vi "Chamber controller March 30 2017.vi"() -> ()   [LabVIEW 2014]
uses:
  <vilib>/Instr/_visa.llb/VISA Configure Serial Port (Instr).vi
  Environmental Chamber LabVIEW and Instruments/Drivers and Software/Keithley 2100 Series/Public/Configure/Configure 2 Wire Resistance.vi
  <vilib>/Utility/file.llb/Write To Spreadsheet File (string).vi
  <vilib>/Utility/file.llb/Read From Spreadsheet File (string).vi
  Environmental Chamber LabVIEW and Instruments/Drivers and Software/keithley_6430/Keithley 6430/Public/Data/Read (Single Point).vi
  Environmental Chamber LabVIEW and Instruments/Drivers and Software/LabVIEW 8.2 Drivers/keithley_24xx/Keithley 24XX/Public/Data/Read (Single Point).vi
  Environmental Chamber LabVIEW and Instruments/Drivers and Software/keithley_24xx/Keithley 24XX/Keithley 24XX.lvlib
  Environmental Chamber LabVIEW and Instruments/Drivers and Software/keithley_6430/Keithley 6430/Keithley 6430.lvlib
  Environmental Chamber LabVIEW and Instruments/Drivers and Software/Keithley 2100 Series/Keithley 2100 Series.lvlib
panel:
  in  "points":i32=10
  in  "average points?":bool
  in  "Pressure parameters cluster":T1={"valve % open"=0.0, "Desired pressure"=0.0, "Vapor sccm"=0.0, "Gas sccm"=0.0, "Valve mode"=enum."% Open", "Pressure Mode"=enum."Abs. pressure", "analyte partial pressure"=23.8, "Turbo pump\nauto on"=TRUE, "Valve position (%)"=0.0, "read pressure"=0.0, "read vapor flow"=0.0, "read gas flow"=0.0} caption="Pressure settings" {"read gas flow" format="%#_3g"; "read vapor flow" format="%#_3g"; "read pressure" format="%#_7f"; "Valve position (%)" format="%#_3g"; "analyte partial pressure" min=0.0 max=100.0 step=5.0; "Gas sccm" min=0 max=200 step=5; "Vapor sccm" min=0 max=200 step=5; "Desired pressure" min=0.0 max=760.0 step=5.0; "valve % open" min=0.0 max=100.0 step=5.0 format="%#_2f"}
  out "pressure chart":cluster{"pressure":dbl}(graph)
  out "arduino qcm stack plot":T2(graph)
  in  "K-2420 tab control":enum32{"K-2420 Measure", "K-2420 Apply bias"}(tab)
  out "K-2420 2":cluster{"Resistance":sgl}(graph)
  in  "Bias (V)":dbl min=-5.0 max=5.0 step=5e-06
  out "K-2420 4":cluster{"Applied Voltage (V)":dbl}(graph)
  out "saving data?":bool
  in  "Data logging settings":T3={"Save during sequence only"=TRUE, "Save now"=FALSE, "sec between points"=0.0, "Current data file path"=path "", "Save sample/gas names"={"QCM1"="", "QCM2"="", "QCM3"="", "QCM4"="", "QCM5"="NOT WORKING", "QCM6"="", "SRS"="bareAu", "K-2420"="", "K-6430"="", "K-2100"="", "Gas"="NOT WORKING", "Vapor"="CO2"}, "add notes to file"=FALSE} {"sec between points" min=0.0 max=30.0 format="%#_13g"}
  in  "Sequence cluster":T4={"Save sequence"=FALSE, "Clear sequence"=FALSE, "Import sequence file"=FALSE, "Run Sequence"=FALSE, "Stop program when sequence ends"=TRUE, "User-defined\nsequence"=[], "Sequence end time"="", "Sequence\npreview"=[], "Current\nstep"=0, "Display"=0, "Sequence length (hrs)"=0.0} caption="Pressure settings" {"Display" items=["pressure", "gas flow", "vapor flow", "bias"]}
  out "J-KEM temp chart":dbl(graph)
  out "State date/time":string caption="Start time"
  out "K-2100 (Ohm)":cluster{"Measurement":dbl}(graph) caption="K-2100"
  out "K-6430":cluster{"Measurement":dbl}(graph)
  in  "Gate time (s)":enum16{"0.1", "1.0 ", "10"}(ring)=enum."1.0 "
  out "Hz":dbl format="%#.7f"
  out "QCM plot":T5(graph)
  in  "Stop":bool
  in  "Clear all charts":bool
  out "O2 sensor output":dbl[](array[numeric]) caption="atm\nTorr"
  in  "rapidox O2 Sensor":bool
  in  "setnag O2 Pump":bool
  in  "Baud Rate 2":i32(ring)=2 items=["2400", "4800", "9600", "19200", "38400", "57600", "115200"]
  in  "Com Port":i32(ring) items=["Com 1", "Com 2", "Com 3", "Com 4", "Com 5", "Com 6", "COM 7", "COM 8", "COM 9", "COM 10", "COM 11", "COM 12", "com 13", "COM 14"]
  in  "Com Port 2":i32(ring) items=["Com 1", "Com 2", "Com 3", "Com 4", "Com 5", "Com 6", "COM 7", "COM 8", "COM 9", "COM 10", "COM 11", "COM 12", "com 13", "COM 14"]
  out "Waveform Chart":cluster{dbl}(graph)
  out "O2 Concentration (PPM)":dbl
  out "Waveform Chart 6":cluster{dbl}(graph)
  # "SRS"
  # "Currently Unused"
  # "100%"
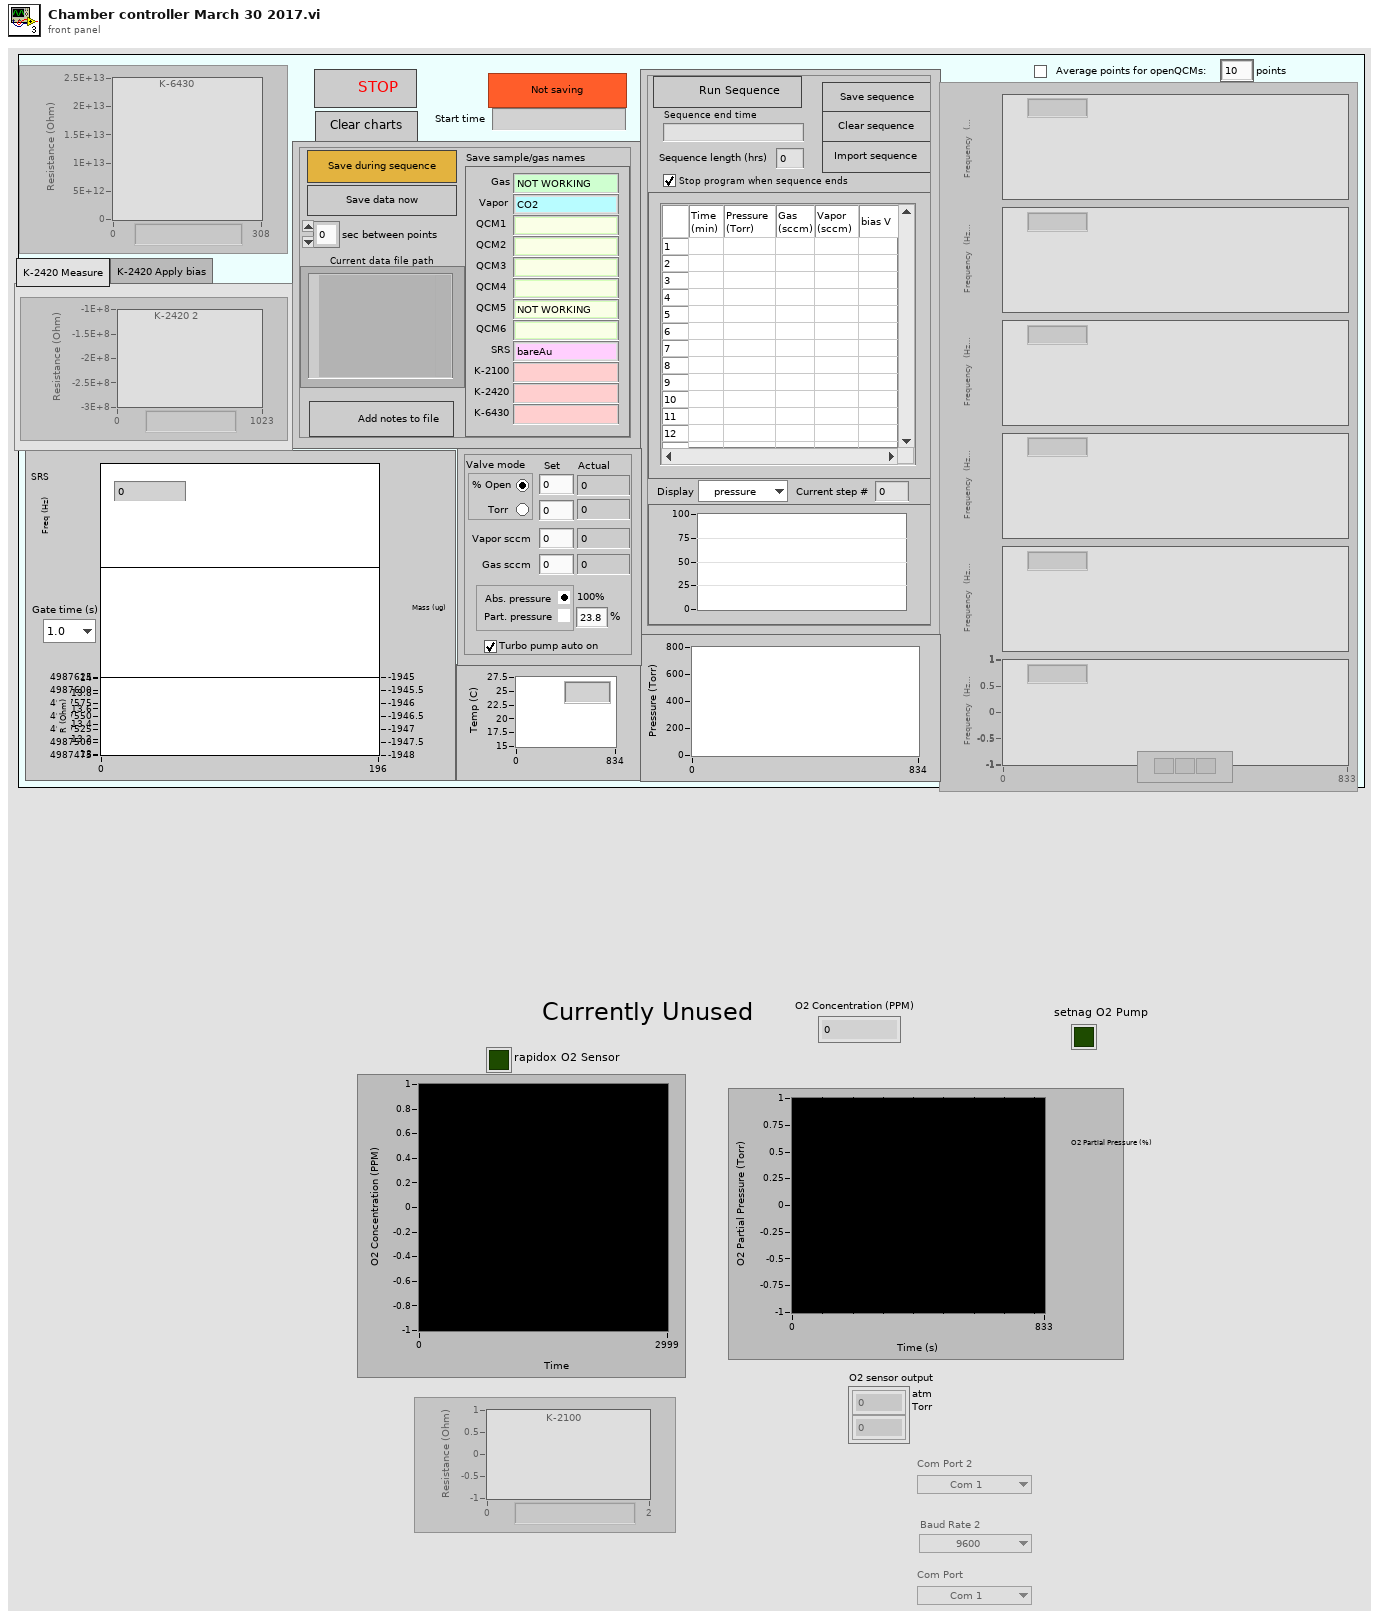
[diagram p1: front panel]
types:
  T1 = cluster{"valve % open":dbl, "Desired pressure":dbl, "Vapor sccm":sgl, "Gas sccm":sgl, "Valve mode":enum32{"% Open", "Torr "}, "Pressure Mode":enum32{"Abs. pressure", " Part. pressure"}, "analyte partial pressure":dbl, "Turbo pump\nauto on":bool, "Valve position (%)":dbl, "read pressure":dbl, "read vapor flow":dbl, "read gas flow":dbl}
  T2 = cluster{"mean":dbl, "mean":dbl, "mean":dbl, "mean":dbl, "mean":dbl, "mean":dbl}
  T3 = cluster{"Save during sequence only":bool, "Save now":bool, "sec between points":dbl, "Current data file path":path, "Save sample/gas names":cluster{"QCM1":string, "QCM2":string, "QCM3":string, "QCM4":string, "QCM5":string, "QCM6":string, "SRS":string, "K-2420":string, "K-6430":string, "K-2100":string, "Gas":string, "Vapor":string}, "add notes to file":bool}
  T4 = cluster{"Save sequence":bool, "Clear sequence":bool, "Import sequence file":bool, "Run Sequence":bool, "Stop program when sequence ends":bool, "User-defined\nsequence":string[][], "Sequence end time":string, "Sequence\npreview":cluster{dbl[], dbl[]}[], "Current\nstep":i32, "Display":u16, "Sequence length (hrs)":dbl}
  T5 = cluster{"Frequency out":dbl, "Numeric Control":dbl, "Resistance out":dbl}
  T6 = cluster{"Keithley 6430":bool, "J-KEM":bool, "Keithley 2420":bool, "Keithley 2100":bool, "SRS QCM":bool, "Pressure control":bool, "Arduino":bool}
  T7 = cluster{"Arduino 1":refnum<visa-resource-name>, "Arduino 2":refnum<visa-resource-name>, "Arduino 3":refnum<visa-resource-name>, "Arduino 4":refnum<visa-resource-name>, "Arduino 5":refnum<visa-resource-name>, "Arduino 6":refnum<visa-resource-name>}
  T8 = enum8{"Enabled", "Disabled", "Disabled and Grayed Out"}
  T9 = enum16{"open", "open or create", "create or replace", "create", "open (read only)"}
  T10 = enum16{"no parity", "odd parity", "even parity", "mark parity", "space parity"}
  T11 = cluster{"mean":dbl, "mean":dbl, "mean":dbl, "mean":dbl, "mean":dbl, "mean":dbl}[]
  T12 = cluster{"Frequency out":dbl, "Numeric Control":dbl, "Resistance out":dbl}[]
  T13 = cluster{"String":string, "String":string, "String":string}
  T14 = cluster{bool, "task out":refnum<k21>, "error out":errorcluster, "task out":refnum<k21>, "error out":errorcluster, "turbo pump":refnum<visa-resource-name>, "error out":errorcluster}
  T15 = cluster{bool, "task out":refnum<k21>, "error out":errorcluster, "task out":refnum<k21>, "error out":errorcluster, "VISA resource name out":refnum<visa-resource-name>, "error out":errorcluster}
  T16 = cluster{bool, "VISA resource name":refnum<visa-resource-name>, "error out":errorcluster}
  T17 = cluster{bool, "VISA resource name out":refnum<visa-resource-name>, "error out":errorcluster}
  T18 = cluster{"VISA resource name out":refnum<visa-resource-name>, "error out":errorcluster, "VISA resource name out":refnum<visa-resource-name>, "error out":errorcluster, "VISA resource name out":refnum<visa-resource-name>, "error out":errorcluster, "VISA resource name out":refnum<visa-resource-name>, "error out":errorcluster, "VISA resource name out":refnum<visa-resource-name>, "error out":errorcluster, "VISA resource name out 2":refnum<visa-resource-name>, "error out 2":errorcluster}
  T19 = cluster{"Boolean":bool, "VISA resource name out":refnum<visa-resource-name>, "error out":errorcluster}
  T20 = cluster{bool, "VISA out":refnum<visa-resource-name>, "error out":errorcluster}
  T21 = cluster{"Boolean":bool, "VISA out":refnum<visa-resource-name>, "error out":errorcluster}
  T22 = cluster{"Numeric Control":dbl, "Cluster":cluster{"Numeric Control":dbl}, "String":string, "error out":errorcluster}
  T23 = cluster{bool, "Com Port":i32, "Numeric Control out":dbl}
  T24 = cluster{"Arduino address":refnum<visa-resource-name>, "error in (no error)":errorcluster, "Arduino address 2":refnum<visa-resource-name>, "error in (no error) 2":errorcluster, "Arduino address 3":refnum<visa-resource-name>, "error in (no error) 3":errorcluster, "Arduino address 4":refnum<visa-resource-name>, "error in (no error) 4":errorcluster, "Arduino address 5":refnum<visa-resource-name>, "error in (no error) 5":errorcluster, "Arduino address 6":refnum<visa-resource-name>, "error in (no error) 6":errorcluster}
  T25 = cluster{"String":string, "String":string, "String":string, "String":string, "String":string, "String":string}
  T26 = cluster{"valve % open":dbl, "Desired pressure":dbl, "Vapor sccm":sgl, "Gas sccm":sgl, "Valve mode":enum32{"% Open", "Torr "}, "Pressure Mode":enum32{"Abs. pressure", " Part. pressure"}, "analyte partial pressure":dbl}
  T27 = cluster{"User-defined\nsequence":string[][], "Present (s)":dbl, "current  step # in":i32, "sequence end time in":timestamp}
  T28 = cluster{"current  step # in":i32, "sequence end time in":timestamp, "Boolean":bool}
  T29 = cluster{"press/RH/gas/vapor":cluster{"pressure":string, "RH":string, "gas flow":string, "vapor flow":string}, "Cluster":cluster{"Valve position (%)":dbl, "read pressure":dbl, "read vapor flow":dbl, "read gas flow":dbl}}
  T30 = cluster{"Boolean":bool, "task out":refnum<k21>, "error out":errorcluster, "task out":refnum<k21>, "error out":errorcluster, "VISA resource name out":refnum<visa-resource-name>, "error out":errorcluster}
  T31 = cluster{"String":dbl, "String":dbl, "String":dbl, "String":dbl, "String":dbl, "String":dbl}
  T32 = cluster{"pressure":string, "RH":string, "gas flow":string, "vapor flow":string}
  T33 = cluster{"Valve position (%)":dbl, "read pressure":dbl, "read vapor flow":dbl, "read gas flow":dbl}
  T34 = cluster{"f":dbl, "f":dbl, "f":dbl, "f":dbl, "f":dbl}[]
  T35 = cluster{"QCM1":string, "QCM2":string, "QCM3":string, "QCM4":string, "QCM5":string, "QCM6":string, "SRS":string, "K-2420":string, "K-6430":string, "K-2100":string, "Gas":string, "Vapor":string}
  T36 = cluster{"String data out":string, string, string, string}
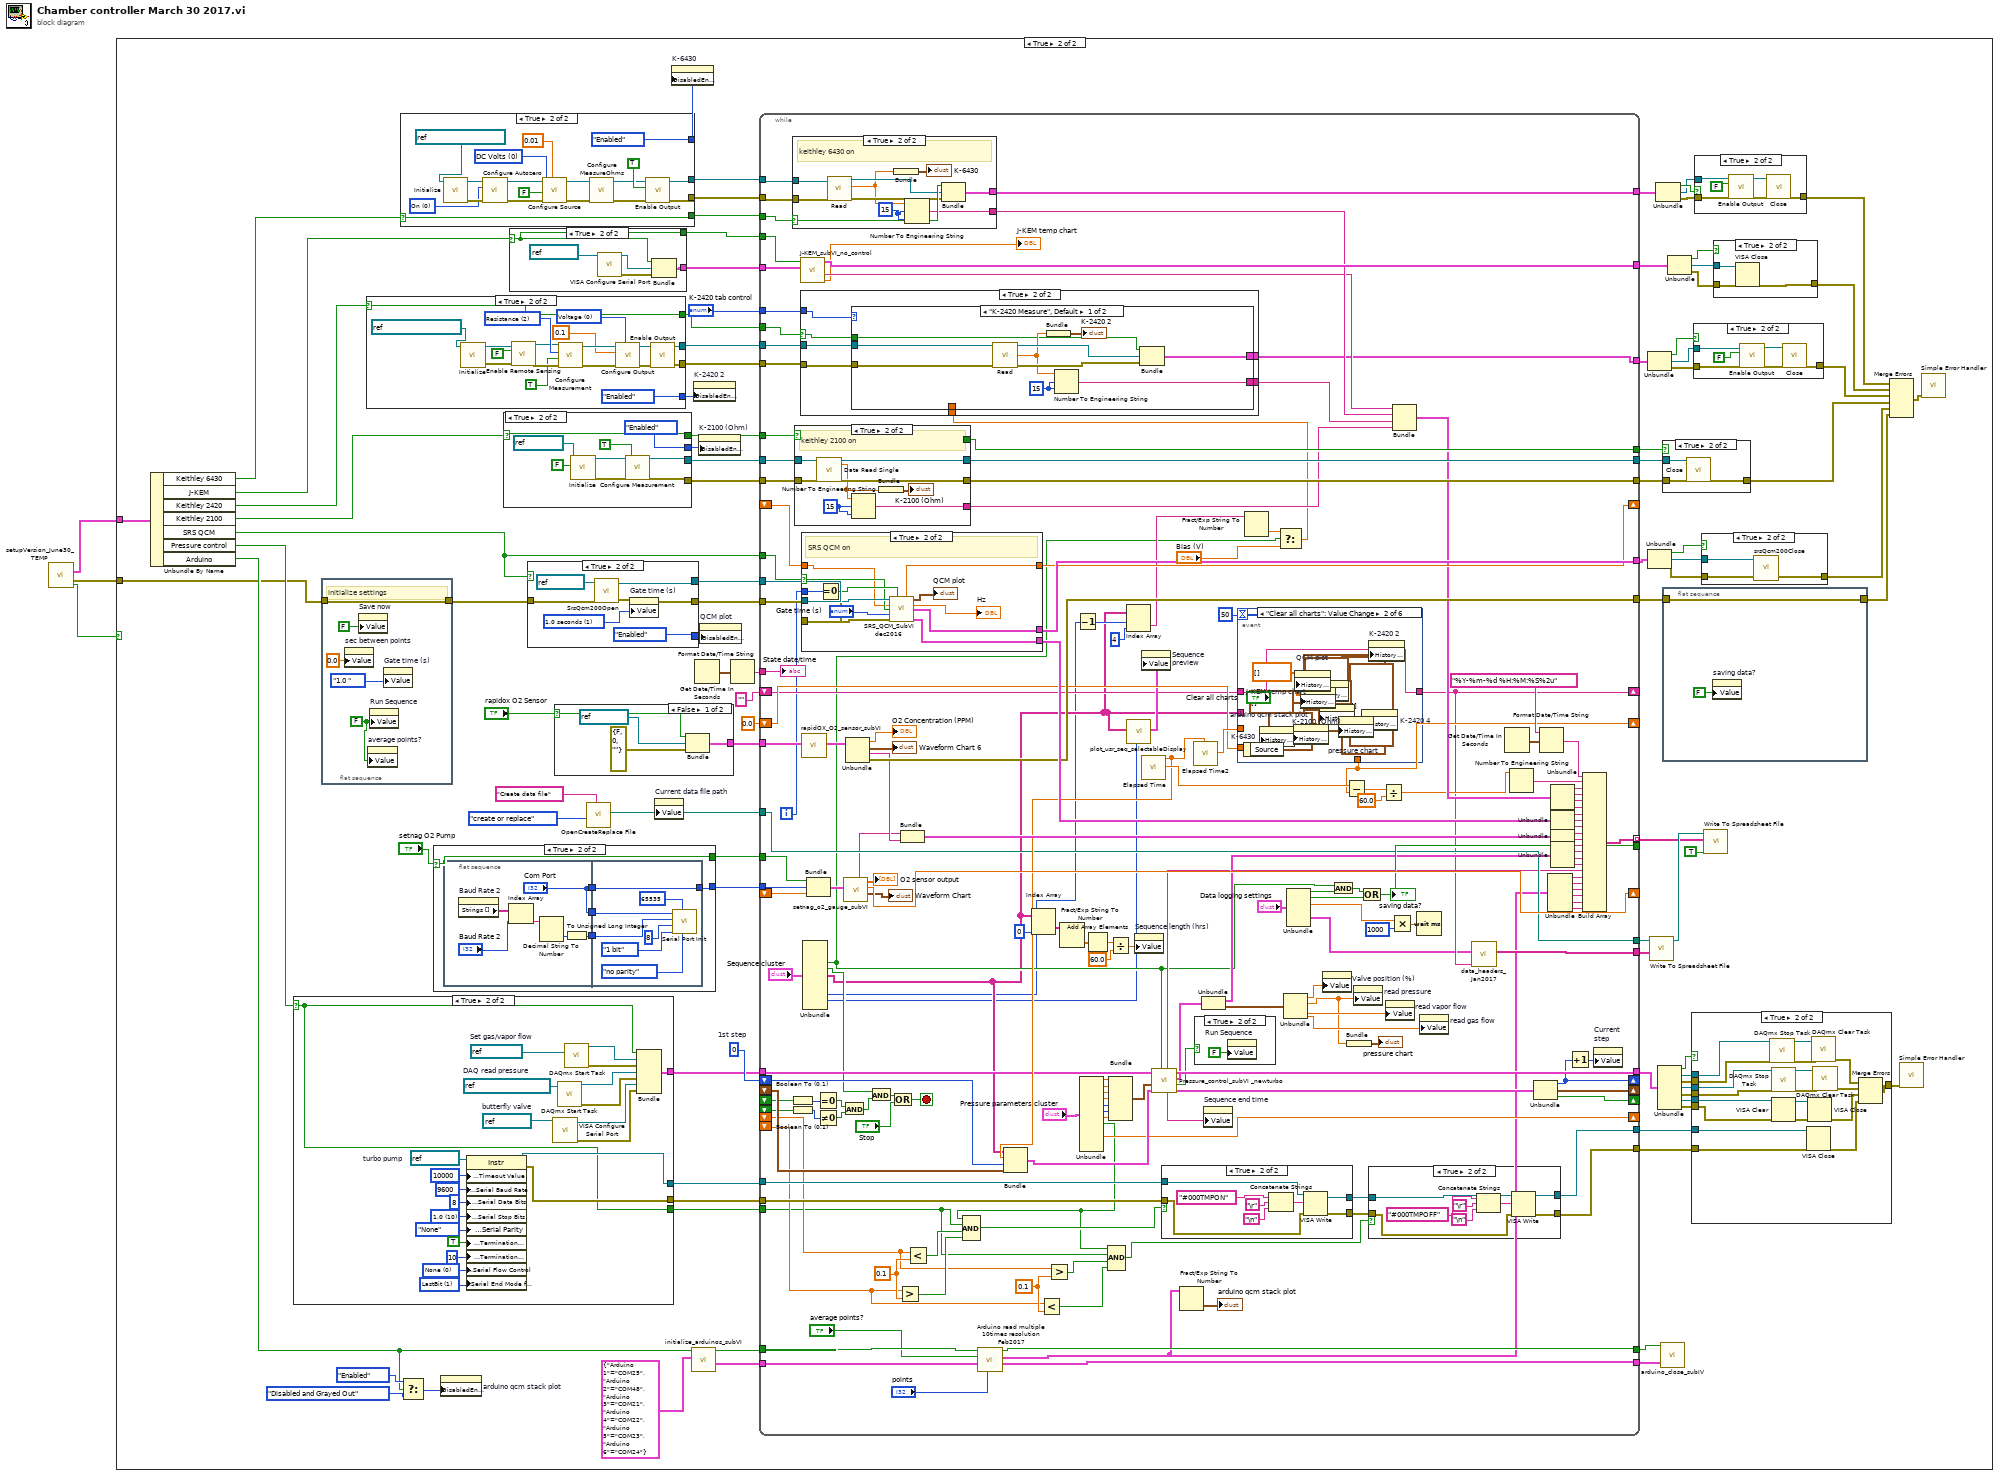
[diagram p0: block diagram]
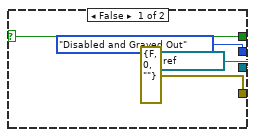
[diagram p4: hidden frame]
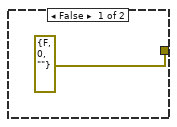
[diagram p5: hidden frame]
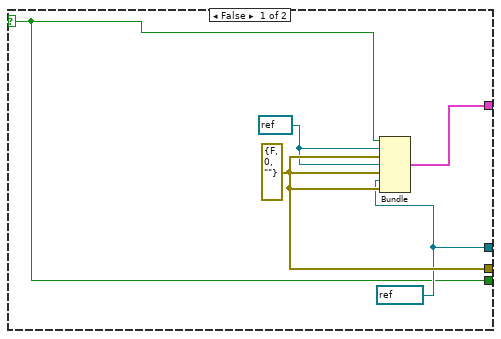
[diagram p6: hidden frame]
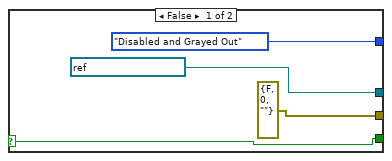
[diagram p8: hidden frame]
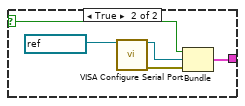
[diagram p9: hidden frame]
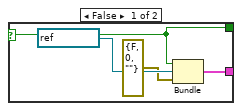
[diagram p11: hidden frame]
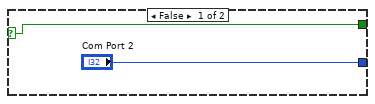
[diagram p12: hidden frame]
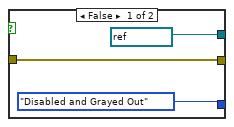
[diagram p14: hidden frame]
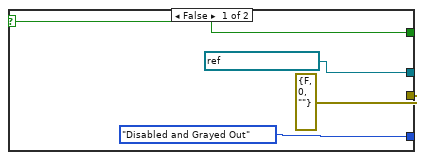
[diagram p16: hidden frame]
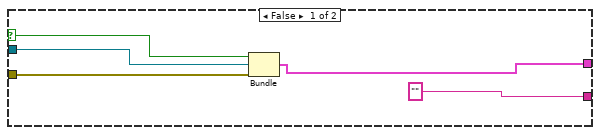
[diagram p17: hidden frame]
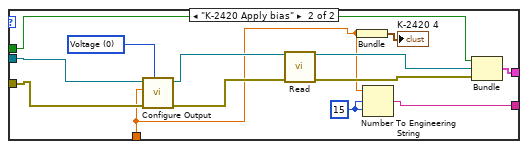
[diagram p18: hidden frame]
diagram:
  n1 = call "setupVersion_June30_TEMP.vi"() -> ("Instruments on/off"=w1:T6, "error IO"=w2:errorcluster, "OK"=w3:bool)  [unwired: 13 in]
  n2 = case shown="True" w3 {
    tunnel: w2 -> [_ w22]
    tunnel: w1 -> [_ w32]
    frame False {
    }
    frame True {
      w38 = 0  # 1st step
      n3 = Unbundle By Name(w32) -> ("Keithley 6430"=w31:bool, "J-KEM"=w30:bool, "Keithley 2420"=w29:bool, "Keithley 2100"=w28:bool, "SRS QCM"=w27:bool, "Pressure control"=w26:bool, "Arduino"=w25:bool)
      n4 = case shown="True" w26 {
        selector: w26 -> [w144 w149]
        tunnel: [w148 w150] -> w20
        tunnel: [w147 w152] -> w12
        tunnel: [w145 w151] -> w13
        tunnel: [w144 w149] -> w11
        frame False {
          w145 = refnum<visa-resource-name> refnum ("turbo pump")
          w146 = refnum<k21> refnum ("task out")
          w147 = errorcluster {"status"=FALSE, "code"=0, "source"=""} ("error out")
          n5 = Bundle(w144, "task out"=w146, "error out"=w147, "task out"=w146, "error out"=w147, "turbo pump"=w145, "error out"=w147) -> (w148:T14)  [unwired: 1 in]
        }
        frame True {
          w156 = u16 1 items=["None", "LastBit", "TermChar"] ("Serial Settings:Serial End Mode for Reads")
          w154 = u16 0 items=["None", "XON/XOFF", "RTS/CTS", "XON/XOFF & RTS/CTS", "DTR/DSR", "XON/XOFF & DTR/DSR"] ("flow control (0:none)")
          w157 = u16 10 items=["1.0"=10, "1.5"=15, "2.0"=20] ("stop bits (10: 1 bit)")
          w153 = refnum<visa-resource-name> "COM7"  # turbo pump
          w169 = refnum<visa-resource-name> "COM5"  # butterfly valve
          w170 = refnum<k21> "Setflow"  # Set gas/vapor flow
          w171 = refnum<k21> "AllDaqReadings"  # DAQ read pressure
          n6 = property class="Instr"(reference=w153, "General Settings:Timeout Value"=u32 10000 ("timeout (10sec)"), "Serial Settings:Serial Baud Rate"=u32 9600 ("baud rate (9600)"), "Serial Settings:Serial Data Bits"=u16 8 ("data bits (8)"), "Serial Settings:Serial Stop Bits"=w157, "Serial Settings:Serial Parity"=enum16{"None", "Odd", "Even", "Mark", "Space"}."None" ("parity (0:none)"), "Message Based Settings:Termination Character Enable"=TRUE ("Enable Termination\nChar (T)"), "Message Based Settings:Termination Character"=u8 10 ("termination char\n(0xA = '\\n' = LF)"), "Serial Settings:Serial Flow Control"=w154, "Serial Settings:Serial End Mode for Reads"=w156) -> (reference out=w151:refnum<visa-resource-name>, error out=w152:errorcluster)  [unwired: 1 in]
          n7 = call-poly "VISA Configure Serial Port"("VISA resource name"=w169) -> ("VISA resource name out"=w164:refnum<visa-resource-name>, "error out"=w163:errorcluster)  [unwired: 13 in]
          n8 = call <vilib>:"DAQmx Start Task.vi"("task/channels in"=w171) -> ("task out"=w166:refnum<k21>, "error out"=w165:errorcluster)  [unwired: 13 in]
          n9 = call <vilib>:"DAQmx Start Task.vi"("task/channels in"=w170) -> ("task out"=w168:refnum<k21>, "error out"=w167:errorcluster)  [unwired: 13 in]
          n10 = Bundle(w149, "task out"=w168, "error out"=w167, "task out"=w166, "error out"=w165, "VISA resource name out"=w164, "error out"=w163) -> (w150:T15)  [unwired: 1 in]
        }
      }
      n11 = flat-sequence {
        tunnel: [w101] -> w21
        tunnel: w22 -> [w101]
        frame #0 {
          w100 = FALSE ("Value")
          # "initialize settings"
          n12 = property on="sec between points" class="DigNum (strict)"("Value"=0.0) -> ()  [unwired: 2 in, 2 out]
          n13 = property on="Save now" class="Bool (strict)"("Value"=FALSE) -> ()  [unwired: 2 in, 2 out]
          n14 = property on="average points?" class="Bool (strict)"("Value"=w100) -> ()  [unwired: 2 in, 2 out]
          n15 = property on="Run Sequence" class="Bool (strict)"("Value"=w100) -> ()  [unwired: 2 in, 2 out]
          n16 = property on="Gate time (s)" class="Enum (strict)"("Value"=enum16{"0.1", "1.0 ", "10"}."1.0 " ("Gate time (sec)")) -> ()  [unwired: 2 in, 2 out]
        }
      }
      n17 = case shown="True" w29 {
        selector: w29 -> [w264 w268]
        tunnel: [refnum<visa-resource-name> "GPIB1::24::INSTR" ("VISA resource name") w277] -> w97
        tunnel: [errorcluster {"status"=FALSE, "code"=0, "source"=""} ("error out") w272] -> w96
        tunnel: [T8."Disabled and Grayed Out" ("Disabled") T8."Enabled" ("Disabled")] -> w4
        tunnel: [w264 w268] -> w54
        frame False {
        }
        frame True {
          w279 = u16 0 items=["Voltage", "Current"] ("Source Mode  (0: Voltage)")
          w284 = u16 2 items=["Volts", "Current", "Resistance"] ("Function (0: Volts)")
          n18 = call "Initialize.vi"("VISA resource name"=refnum<visa-resource-name> "GPIB1::24::INSTR") -> ("error out"=w273:errorcluster, "VISA resource name out"=w276:refnum<visa-resource-name>)  [unwired: 9 in]
          n19 = call "Enable Remote Sensing.vi"("error in (no error)"=w273, "Enable Remote Sensing (T: Enable)"=FALSE ("4-wire?"), "VISA resource name"=w276) -> ("error out"=w274:errorcluster, "VISA resource name out"=w275:refnum<visa-resource-name>)  [unwired: 7 in]
          n20 = call "Configure Measurement.vi"("error in (no error)"=w274, "Enable Auto Range (T:Enable)"=TRUE, "Function (0: Volts)"=w284, "VISA resource name"=w275) -> ("error out"=w283:errorcluster, "VISA resource name out"=w282:refnum<visa-resource-name>)  [unwired: 6 in]
          n21 = call "Configure Output.vi"("Source Mode  (0: Voltage)"=w279, "error in (no error)"=w283, "Output Level (0)"=0.1 ("Applied Voltage (V)"), "VISA resource name"=w282) -> ("error out"=w281:errorcluster, "VISA resource name out"=w280:refnum<visa-resource-name>)  [unwired: 6 in]
          n22 = call "Enable Output.vi"("error in (no error)"=w281, "VISA resource name"=w280) -> ("error out"=w272:errorcluster, "VISA resource name out"=w277:refnum<visa-resource-name>)  [unwired: 8 in]
        }
      }
      n23 = case shown="True" w31 {
        selector: w31 -> [w179 w184]
        tunnel: [refnum<visa-resource-name> "GPIB0::29::INSTR" ("VISA resource name") w195] -> w66
        tunnel: [errorcluster {"status"=FALSE, "code"=0, "source"=""} ("error out") w196] -> w65
        tunnel: [T8."Disabled and Grayed Out" ("Disabled") T8."Enabled" ("Disabled")] -> w60
        tunnel: [w179 w184] -> w53
        frame False {
        }
        frame True {
          w185 = u16 0 items=["DC Volts", "DC Current"] ("Source Function (0: DC Volts)")
          w192 = u16 0 items=["On", "Off", "Once"] ("Autozero  (0: On)")
          n24 = call "Initialize.vi"("VISA resource name"=refnum<visa-resource-name> "GPIB2::19::INSTR") -> ("error out"=w193:errorcluster, "VISA resource name out"=w194:refnum<visa-resource-name>)  [unwired: 4 in, 5 out]
          n25 = call "Configure Autozero.vi"("error in (no error)"=w193, "Autozero  (0: On)"=w192, "VISA resource name"=w194) -> ("error out"=w188:errorcluster, "VISA resource name out"=w190:refnum<visa-resource-name>)  [unwired: 7 in]
          n26 = call "Configure Source.vi"("V-Source Level [V]"=0.01, "error in (no error)"=w188, "Auto Range (T:Enable)"=FALSE, "Source Function (0: DC Volts)"=w185, "VISA resource name"=w190) -> ("error out"=w187:errorcluster, "VISA resource name out"=w189:refnum<visa-resource-name>)  [unwired: 5 in]
          n27 = call "Configure MeasureOhms.vi"("error in (no error)"=w187, "VISA resource name"=w189) -> ("error out"=w200:errorcluster, "VISA resource name out"=w198:refnum<visa-resource-name>)  [unwired: 4 in, 4 out]
          n28 = call "Enable Output.vi"("error in (no error)"=w200, "Enable Output (F:Off)"=TRUE ("Output (F:Off)"), "VISA resource name"=w198) -> ("error out"=w196:errorcluster, "VISA resource name out"=w195:refnum<visa-resource-name>)  [unwired: 7 out]
        }
      }
      n29 = Select(t=T8."Enabled" ("Disabled"), s=w25, f=T8."Disabled and Grayed Out" ("Disabled")) -> (s? t:f=w6:T8)
      n30 = case shown="True" "setnag O2 Pump" {
        selector: "setnag O2 Pump" -> [w223 w225]
        tunnel: ["Com Port 2" w226] -> w93
        tunnel: [w223 w225] -> w43
        frame False {
        }
        frame True {
          n31 = flat-sequence {
            tunnel: ["Com Port"] -> w229
            tunnel: [w231] -> w228
            tunnel: ["Com Port"] -> w227
            tunnel: w229 -> [w237]
            tunnel: w228 -> [w236]
            tunnel: w227 -> [w238]
            tunnel: [w238] -> w226
            frame #0 {
              n32 = property on="Baud Rate 2" class="Ring (strict)"() -> ("Strings []"=w233:string[])  [unwired: 2 in, 2 out]
              n33 = Index Array(array=w233, index="Baud Rate 2") -> (element=w234:string)
              n34 = Decimal String To Number(string=w234) -> (number=w232:i32)  [unwired: 2 in, 1 out]
              n35 = To Unsigned Long Integer(number=w232) -> (unsigned 32bit integer=w231:u32)
            }
            frame #1 {
              n36 = call <vilib>:"Serial Port Init.vi"("parity"=T10."no parity", "buffer size"=u16 65535, "stop bits"=enum16{"1 bit", "1.5 bits", "2 bits"}."1 bit", "data bits"=u16 8, "baud rate"=w236, "port number"=w237) -> ()  [unwired: 1 in, 1 out]
            }
          }
        }
      }
      n37 = property on="arduino qcm stack plot" class="WFChart (strict)"("DisabledEnum"=w6) -> ()  [unwired: 2 in, 2 out]
      n38 = case shown="True" w28 {
        selector: w28 -> [w112 w117]
        tunnel: [refnum<visa-resource-name> "K-2100" ("VISA resource name out") w120] -> w52
        tunnel: [errorcluster {"status"=FALSE, "code"=0, "source"=""} ("error out") w119] -> w51
        tunnel: [w112 w117] -> w50
        tunnel: [T8."Disabled and Grayed Out" ("Disabled") T8."Enabled" ("Disabled")] -> w45
        frame False {
        }
        frame True {
          n39 = call "Initialize.vi"("VISA resource name"=refnum<visa-resource-name> "K-2100", "Reset? (T: Reset)"=FALSE) -> ("VISA resource name out"=w121:refnum<visa-resource-name>, "error out"=w118:errorcluster)  [unwired: 16 in]
          n40 = call-poly "Configure Measurement.vi"("VISA resource name"=w121, "error in (no error)"=w118, "Auto Range? (T: Auto)"=TRUE) -> ("VISA resource name out"=w120:refnum<visa-resource-name>, "error out"=w119:errorcluster)  [unwired: 15 in]
        }
      }
      n41 = case shown="True" w30 {
        selector: w30 -> [w214 w219]
        tunnel: [w215 w220] -> w82
        tunnel: [w214 w219] -> w76
        frame False {
          n42 = Bundle(w214, "VISA resource name"=refnum<visa-resource-name> "COM3", "error out"=errorcluster {"status"=FALSE, "code"=0, "source"=""}) -> (w215:T16)  [unwired: 1 in]
        }
        frame True {
          n43 = call-poly "VISA Configure Serial Port"("VISA resource name"=refnum<visa-resource-name> "COM3") -> ("VISA resource name out"=w221:refnum<visa-resource-name>, "error out"=w218:errorcluster)  [unwired: 13 in]
          n44 = Bundle(w219, "VISA resource name out"=w221, "error out"=w218) -> (w220:T17)  [unwired: 1 in]
        }
      }
      n45 = case shown="True" w27 {
        tunnel: [refnum<visa-resource-name> "COM6" ("VISA in") w253] -> w95
        tunnel: [w248 w250] -> w94
        tunnel: w21 -> [w248 w255]
        tunnel: [T8."Disabled and Grayed Out" ("Disabled") T8."Enabled" ("Disabled")] -> w61
        frame False {
        }
        frame True {
          w252 = u16 1 items=["0.1 seconds", "1.0 seconds", "10.0 seconds"] ("Gate time")
          n46 = call "SrsQcm200Open.vi"("error in"=w255, "VISA in"=refnum<visa-resource-name> "COM6") -> ("error out"=w251:errorcluster, "VISA out"=w253:refnum<visa-resource-name>)  [unwired: 3 in]
          n47 = property on="Gate time (s)" class="Enum (strict)"(error in=w251, "Value"=w252) -> (error out=w250:errorcluster)  [unwired: 1 in, 1 out]
        }
      }
      n48 = case shown="False" "rapidox O2 Sensor" {
        selector: "rapidox O2 Sensor" -> [w201 w206]
        tunnel: [w202 w207] -> w72
        frame False {
          n49 = Bundle(w201, "VISA resource name"=refnum<visa-resource-name> "COM7", "error out"=errorcluster {"status"=FALSE, "code"=0, "source"=""}) -> (w202:T16)  [unwired: 1 in]
        }
        frame True {
          n50 = call-poly "VISA Configure Serial Port"("VISA resource name"=refnum<visa-resource-name> "COM7") -> ("VISA resource name out"=w208:refnum<visa-resource-name>, "error out"=w205:errorcluster)  [unwired: 13 in]
          n51 = Bundle(w206, "VISA resource name out"=w208, "error out"=w205) -> (w207:T17)  [unwired: 1 in]
        }
      }
      n52 = call "OpenCreateReplace File.vi"("prompt"="Create data file", "function (open:0)"=T9."create or replace") -> ("new file path"=w8:path)  [unwired: 6 in, 3 out]
      n53 = property on="Current data file path" class="Path"("Value"=w8) -> ()  [unwired: 2 in, 2 out]
      n54 = property on="K-6430" class="WFChart (strict)"("DisabledEnum"=w60) -> ()  [unwired: 2 in, 2 out]
      n55 = call "initialize_arduinos_subVI.vi"("arduino 1-6 addresses"=T7 {"Arduino 1"="COM25", "Arduino 2"="COM48", "Arduino 3"="COM21", "Arduino 4"="COM22", "Arduino 5"="COM23", "Arduino 6"="COM24"} ("Arduino COMs"), "arduinos on?"=w25) -> ("arduino addresses/errors"=w39:T18, "arduinos on/off"=w58:bool)  [unwired: 8 in]
      n56 = property on="K-2420 2" class="WFChart (strict)"("DisabledEnum"=w4) -> ()  [unwired: 2 in, 2 out]
      n57 = Get Date/Time In Seconds() -> (seconds since 1Jan1904=w99:timestamp)
      n58 = property on="K-2100 (Ohm)" class="WFChart (strict)"("DisabledEnum"=w45) -> ()  [unwired: 2 in, 2 out]
      n59 = property on="QCM plot" class="WFChart (strict)"("DisabledEnum"=w61) -> ()  [unwired: 2 in, 2 out]
      n60 = Format Date/Time String(seconds (now)=w99) -> (date/time string=w42:string)  [unwired: 2 in]
      n61 = while {
        shift-right: [w464] -> _
        shift-left: _ -> [w405]
        tunnel: [w452] -> w59 mode=indexing if=w426
        tunnel: w54 -> [w325]
        tunnel: w97 -> [w327]
        tunnel: w96 -> [w326]
        tunnel: w95 -> [w463]
        tunnel: w94 -> [w462]
        tunnel: w27 -> [w461]
        tunnel: w43 -> [w407]
        tunnel: w93 -> [w408]
        tunnel: [w320] -> w90
        tunnel: [w460] -> w86
        tunnel: w82 -> [w459]
        tunnel: [w458] -> w81
        tunnel: w76 -> [w457]
        tunnel: w72 -> [w415]
        tunnel: [w411] -> w24
        tunnel: [w356] -> w71
        tunnel: w8 -> [w356]
        shift-right: [w450] -> _
        shift-left: _ -> [w451]
        tunnel: w66 -> [w456]
        tunnel: w65 -> [w455]
        tunnel: [w454] -> w64
        tunnel: [w426] -> _
        tunnel: w58 -> [w298]
        tunnel: w39 -> [w299]
        tunnel: [w296] -> w56
        tunnel: [w295] -> w57
        tunnel: [w300] -> w55
        tunnel: w53 -> [w438]
        tunnel: w52 -> [w425]
        tunnel: w51 -> [w424]
        tunnel: w50 -> [w423]
        tunnel: [w422] -> w49
        tunnel: [w421] -> w48
        tunnel: [w420] -> w47
        shift-right: [w399] -> _
        shift-left: 0.0 ("Elapsed Time (s)") -> [w400]
        tunnel: w42 -> [w390]
        tunnel: w20 -> [w350]
        shift-right: [w353] -> _
        shift-left: w38 -> [w367]
        shift-right: [w372] -> _
        shift-left: _ -> [w370]
        shift-right: [w371] -> _
        shift-left: _ -> [w369]
        shift-left: _ -> [w368]
        tunnel: [w365] -> w37
        tunnel: w13 -> [w345]
        tunnel: w12 -> [w344]
        tunnel: w11 -> [w334]
        tunnel: [w339] -> w10
        tunnel: [w340] -> w9
        shift-right: [w349] -> _
        shift-left: _ -> [w336]
        shift-left: _ -> [w335]
        shift-right: [w302] -> _
        shift-left: "" ("notes to add") -> [w317]
        tunnel: "K-2420 tab control" -> [w304]
        i -> [w303]
        stop <- w428 stop-if-true
        w338 = 0.1 ("y")
        w348 = 0.1 ("y")
        n62 = Boolean To (0,1)(Boolean=w369) -> (0, 1=w436:i16)
        n63 = Boolean To (0,1)(Boolean=w368) -> (0, 1=w435:i16)
        n64 = case "Keithley 6430" shown="True" w438 {
          selector: w438 -> [w554 w565]
          tunnel: w456 -> [w553 w562]
          tunnel: w455 -> [w552 w561]
          tunnel: ["" w564] -> w410
          tunnel: [w551 w563] -> w454
          frame False {
            # "keithley 6430 off"
            n65 = Bundle(w554, "VISA resource name out"=w553, "error out"=w552) -> (w551:T17)  [unwired: 1 in]
          }
          frame True {
            w556 = i16 15 ("width (-)")
            # "keithley 6430 on"
            n66 = call-poly "Read.vi"("error in (no error)"=w561, "VISA resource name"=w562) -> ("error out"=w560:errorcluster, "Measurement"=w558:dbl, "VISA resource name out"=w559:refnum<visa-resource-name>)  [unwired: 1 in, 6 out]
            n67 = Bundle("Measurement"=w558) -> (→"K-6430":cluster{"Measurement":dbl})  [unwired: 1 in]
            n68 = Number To Engineering String(2:w556, 3:w556, 4:w558) -> (0:w564:string)  [unwired: 1 in]
            n69 = Bundle(w565, "VISA resource name out"=w559, "error out"=w560) -> (w563:T17)  [unwired: 1 in]
          }
        }
        n70 = case shown="True" w423 {
          selector: w423 -> [w522 w527]
          tunnel: [w523 w534] -> w421
          tunnel: [w524 w533] -> w420
          tunnel: w425 -> [w523 w532]
          tunnel: w424 -> [w524 w531]
          tunnel: ["" w529] -> w409
          tunnel: [w522 w527] -> w422
          frame False {
            # "keithley 2100 off"
          }
          frame True {
            w526 = i16 15 ("width (-)")
            # "keithley 2100 on"
            n71 = call "Data Read Single.vi"("VISA resource name"=w532, "error in (no error)"=w531) -> ("VISA resource name out"=w534:refnum<visa-resource-name>, "Measurement"=w530:dbl, "error out"=w533:errorcluster)  [unwired: 15 in]
            n72 = Number To Engineering String ("elapsed time (min)")(2:w526, 3:w526, 4:w530) -> (0:w529:string)  [unwired: 1 in]
            n73 = Bundle("Measurement"=w530) -> (→"K-2100 (Ohm)":cluster{"Measurement":dbl})  [unwired: 1 in]
          }
        }
        n74 = call "J-KEM_subVI_no_control.vi"("Address in"=w459, "J-KEM on?"=w457) -> ("Temp (C)"=→"J-KEM temp chart":dbl, "String data out"=w398:string, "Address out"=w458:T19)  [unwired: 6 in, 1 out]
        n75 = case "SRS QCM" shown="True" w461 {
          selector: w461 -> [w568 w578]
          tunnel: w463 -> [w571 w580]
          tunnel: w462 -> [w570 w582]
          tunnel: [w569 w575] -> w460
          tunnel: w451 -> [w566 w576]
          tunnel: [w566 w577] -> w450
          tunnel: [T13 {"String"="", "String"="", "String"=""} ("M,F,MR output cluster") w574] -> w443
          tunnel: w303 -> [_ w583]
          frame False {
            # "SRS QCM off"
            n76 = Bundle(w568, "VISA out"=w571, "error out"=w570) -> (w569:T20)  [unwired: 1 in]
          }
          frame True {
            # "SRS QCM on"
            n77 = Equal To 0?(x=w583) -> (x = 0?=w579:bool)
            n78 = call "SRS_QCM_SubVI  dec2016.vi"("VISA Refnum in"=w580, "first iteration?"=w579, "Frequency  in"=w576, "SRS on?"=w578, "Gate time"="Gate time (s)", "error in (no error)"=w582) -> ("Frequency out 2"=w577:dbl, "freq, mass, MR"=→"QCM plot":T5, "Frequency out"=→"Hz":dbl, "address out"=w575:T21, "M,F,MR output cluster"=w574:T13)  [unwired: 2 in, 3 out]
          }
        }
        n79 = call "rapidOX_O2_sensor_subVI.vi"("rapid ox info in"=w415) -> ("rapidox info out"=w414:T22)  [unwired: 10 in]
        n80 = Unbundle("Sequence cluster") -> ("Run Sequence"=w310:bool, "Stop program when sequence ends"=w309:bool, "User-defined\nsequence"=w308:string[][], "Current\nstep"=w307:i32, "Display"=w306:u16)  [unwired: 6 out]
        n81 = Bundle(w407, "Com Port"=w408, "Numeric Control out"=w405) -> (w406:T23)  [unwired: 1 in]
        n82 = Equal To 0?(x=w436) -> (x = 0?=w433:bool)
        n83 = Not Equal To 0?(x=w435) -> (x != 0?=w434:bool)
        n84 = And(x=w433, y=w434) -> (x .and. y?=w427:bool)
        n85 = call "setnag_o2_gauge_subVI.vi"("setnag info in"=w406) -> ("Cluster"=→"Waveform Chart":cluster{"Numeric Control":dbl}, "Numeric Control out"=w464:dbl, "Array"=→"O2 sensor output":dbl[], "String"=w354:string)  [unwired: 7 in]
        n86 = Unbundle(w414) -> ("Numeric Control"=→"O2 Concentration (PPM)":dbl, "Cluster"=→"Waveform Chart 6":cluster{"Numeric Control":dbl}, "String"=w389:string, "error out"=w411:errorcluster)
        n87 = And(x=w309, y=w427) -> (x .and. y?=w403:bool)
        n88 = Or(x=w403, y="Stop") -> (x .or. y?=w428:bool)
        n89 = Greater?(x=w335, y=w348) -> (0:w347:bool)
        n90 = Bundle("String"=w354, "String"=w389) -> (w388:cluster{"String":string, "String":string})  [unwired: 1 in]
        n91 = Less?(x=w336, y=w348) -> (x < y?=w346:bool)
        n92 = call "Arduino read multiple 10times resolution Feb2017.vi"("# of points to average"="points", "arduino addresses in"=w299, "average points?"="average points?", "arduinos on?"=w298) -> ("arduino addresses out"=w295:T24, "freq out"=w292:T25, "arduinos on"=w296:bool)  [unwired: 4 in]
        n93 = Index Array(array=w308, index (col)=0 ("disabled index (col)")) -> (element=w315:string[])  [unwired: 1 in]
        n94 = Less?(x=w335, y=w338) -> (x < y?=w332:bool)
        n95 = Greater?(x=w336, y=w338) -> (0:w333:bool)
        n96 = Fract/Exp String To Number(string=w315) -> (number=w314:dbl[])  [unwired: 3 in, 1 out]
        n97 = Decrement(x=w307) -> (x-1=w329:i32)
        n98 = Unbundle("Pressure parameters cluster") -> ("valve % open"=w379:dbl, "Desired pressure"=w380:dbl, "Vapor sccm"=w381:sgl, "Gas sccm"=w382:sgl, "Valve mode"=w383:enum32{"% Open", "Torr "}, "Pressure Mode"=w384:enum32{"Abs. pressure", " Part. pressure"}, "analyte partial pressure"=w385:dbl, "Turbo pump\nauto on"=w337:bool, "read pressure"=w349:dbl)  [unwired: 3 out]
        n99 = Compound Arithmetic op=AND(w337, w334, w346, w347) -> (w343:bool)
        n100 = Add Array Elements(numeric array=w314) -> (sum=w313:dbl)
        n101 = Compound Arithmetic op=AND(w337, w334, w333, w332) -> (w331:bool)
        n102 = Divide(x=w313, y=60.0) -> (x/y=w311:dbl)
        n103 = Bundle("valve % open"=w379, "Desired pressure"=w380, "Vapor sccm"=w381, "Gas sccm"=w382, "Valve mode"=w383, "Pressure Mode"=w384, "analyte partial pressure"=w385) -> (w378:T26)  [unwired: 1 in]
        n104 = Index Array(array=w308, index (row)=w329, index (col)=4 ("disabled index (col)")) -> (element=w322:string)
        n105 = call "plot_usr_seq_selectableDisplay.vi"("Display"=w306, "User-defined sequence"=w308) -> ("Sequence Preview"=w328:cluster{dbl[], dbl[]}[])  [unwired: 9 in]
        n106 = property on="Sequence length (hrs)" class="DigNum (strict)"("Value"=w311) -> ()  [unwired: 2 in, 2 out]
        n107 = property on="Sequence\npreview" class="XYGraph (strict)"("Value"=w328) -> ()  [unwired: 2 in, 2 out]
        n108 = call "Elapsed Time"() -> ("Present (s)"=w374:dbl, "Elapsed Time (s)"=w417:dbl)  [unwired: 12 in, 6 out]
        n109 = Bundle("User-defined\nsequence"=w308, "Present (s)"=w374, "current  step # in"=w367, "sequence end time in"=w370) -> (w375:T27)  [unwired: 1 in]
        n110 = call "Pressure_control_subVI _newturbo.vi"("Run Sequence"=w310, "user sequence, present (s) in, current step in, seq time in"=w375, "pressure parameters in"=w378, "pressure control on?/daq IDs/errors"=w350) -> ("current step # out, shift register time out, seq button on?"=w373:T28, "sequence over? USE THIS TO REINITIALIZE RUN SEQUENCE BUTTON SO PROGRAM ENDS"=w364:bool, "save press/RH/gasflow/vaporflow - read valve position/pressure/vaporflow/gasflow"=w363:T29, "pressure control on?/daq IDs/errors out"=w365:T30, "sequence end date/time string"=w366:string, "pressure_setpoint"=w351:string)  [unwired: 2 in]
        n111 = case shown="True" w343 {
          tunnel: w345 -> [w512 w515]
          tunnel: w344 -> [w511 w516]
          tunnel: [w512 w514] -> w342
          tunnel: [w511 w513] -> w341
          frame False {
          }
          frame True {
            n112 = Concatenate Strings("#000TMPON" ("write buffer 2"), "\r", "\n") -> (w517:string)
            n113 = VISA Write(VISA resource name=w515, write buffer=w517, error in (no error)=w516) -> (VISA resource name out=w514:refnum<visa-resource-name>, error out=w513:errorcluster)  [unwired: 1 out]
          }
        }
        n114 = Fract/Exp String To Number(string=w292) -> (number=→"arduino qcm stack plot":T31)  [unwired: 3 in, 1 out]
        n115 = call "Elapsed Time2"("Set Start Time (s)"=w374) -> ("Elapsed Time (s)"=w401:dbl)  [unwired: 11 in, 7 out]
        n116 = case shown="True" w364 {
          frame False {
          }
          frame True {
            n117 = property on="Run Sequence" class="Bool (strict)"("Value"=FALSE ("Run Sequence")) -> ()  [unwired: 2 in, 2 out]
          }
        }
        n118 = Unbundle(w363) -> ("press/RH/gas/vapor"=w362:T32, "Cluster"=w361:T33)
        n119 = property on="Sequence end time" class="Str"("Value"=w366) -> ()  [unwired: 2 in, 2 out]
        n120 = event shown="[1] \"Clear all charts\": Value Change" {
          selector: _ -> [_ _ _ _ _ _]
          dyn-events: _ -> [_ _ _ _ _ _]
          timeout: 50 -> [_ _ _ _ _ _]
          tunnel: w308 -> [_ _ _ _ w548 _]
          tunnel: w401 -> [_ _ _ _ _ _]
          tunnel: w400 -> [w536 _ _ _ _ _]
          tunnel: [w536 _ _ _ _ _] -> w399
          tunnel: [w535 w539 w544 w545 w547 w549] -> w302
          tunnel: w317 -> [w535 w539 w543 w545 w547 w549]
          event Timeout {
            n121 = event-data() -> ()  [unwired: 1 in, 1 out]
          }
          event "Clear all charts": Value Change {
            (unwired) T34 [] ("History Data")
            w537 = cluster{dbl}[] [] ("History Data")
            w542 = cluster{"Resistance":sgl}[] [] ("History Data")
            (unwired) cluster{dbl, "Resistance out":dbl}[] [] ("History Data")
            n122 = event-data() -> ()  [unwired: 1 in, 1 out]
            n123 = property on="K-6430" class="WFChart (strict)"("History Data"=w542) -> ()  [unwired: 2 in, 2 out]
            n124 = property on="Waveform Chart" class="WFChart (strict)"("History Data"=w537) -> ()  [unwired: 2 in, 2 out]
            n125 = property on="QCM plot" class="WFChart (strict)"("History Data"=T12 []) -> ()  [unwired: 2 in, 2 out]
            n126 = property on="K-2100 (Ohm)" class="WFChart (strict)"("History Data"=w542) -> ()  [unwired: 2 in, 2 out]
            n127 = property on="J-KEM temp chart" class="WFChart (strict)"("History Data"=dbl[] []) -> ()  [unwired: 2 in, 2 out]
            n128 = property on="arduino qcm stack plot" class="WFChart (strict)"("History Data"=T11 []) -> ()  [unwired: 2 in, 2 out]
            n129 = property on="pressure chart" class="WFChart (strict)"("History Data"=w537) -> ()  [unwired: 2 in, 2 out]
            n130 = property on="K-2420 4" class="WFChart (strict)"("History Data"=w537) -> ()  [unwired: 2 in, 2 out]
            n131 = property on="K-2420 2" class="WFChart (strict)"("History Data"=w537) -> ()  [unwired: 2 in, 2 out]
          }
          event "Data logging settings.add notes to file": Value Change {
            n132 = event-data() -> ()  [unwired: 1 in, 1 out]
            n133 = call "notes_subVI.vi"("previous notes"=w543) -> ("notes to add"=w544:string)  [unwired: 14 in]
          }
          event "Sequence cluster.Clear sequence": Value Change {
            n134 = event-data() -> ()  [unwired: 1 in, 1 out]
            n135 = property on="User-defined\nsequence" class="Tbl (strict)"("Value"=string[][] []) -> ()  [unwired: 2 in, 2 out]
          }
          event "Sequence cluster.Save sequence": Value Change {
            n136 = event-data() -> ()  [unwired: 1 in, 1 out]
            n137 = call-poly <vilib>:"Write To Spreadsheet File.vi"("2D data"=w548) -> ()  [unwired: 7 in, 1 out]
          }
          event "Sequence cluster.Import sequence file": Value Change {
            n138 = event-data() -> ()  [unwired: 1 in, 1 out]
            n139 = call-poly <vilib>:"Read From Spreadsheet File.vi"() -> ("all rows"=w550:string[][])  [unwired: 7 in, 4 out]
            n140 = property on="User-defined\nsequence" class="Tbl (strict)"("Value"=w550) -> ()  [unwired: 2 in, 2 out]
          }
        }
        n141 = Fract/Exp String To Number(string=w322) -> (number=w321:dbl)  [unwired: 3 in, 1 out]
        n142 = Select(t=w321, s=w310, f="Bias (V)") -> (s? t:f=w324:dbl)
        n143 = case shown="True" w325 {
          selector: w325 -> [w470 w477]
          tunnel: ["" w476] -> w319
          tunnel: [w467 w475] -> w320
          tunnel: w327 -> [w469 w474]
          tunnel: w326 -> [w468 w473]
          tunnel: w324 -> [_ w472]
          tunnel: w304 -> [_ w471]
          frame False {
            n144 = Bundle(w470, "VISA resource name out"=w469, "error out"=w468) -> (w467:T17)  [unwired: 1 in]
          }
          frame True {
            n145 = case shown="\"K-2420 Measure\", Default" w471 {
              tunnel: w474 -> [w482 w494]
              tunnel: w473 -> [w481 w493]
              tunnel: [w480 w491] -> w475
              tunnel: w477 -> [w479 w492]
              tunnel: [w478 w490] -> w476
              tunnel: w472 -> [_ w489]
              frame "K-2420 Measure", Default {
                w483 = i16 15 ("width (-)")
                n146 = call-poly "Read.vi"("VISA resource name"=w482, "error in (no error)"=w481) -> ("VISA resource name out"=w486:refnum<visa-resource-name>, "Resistance"=w484:sgl, "error out"=w485:errorcluster)  [unwired: 7 in, 4 out]
                n147 = Bundle("Resistance"=w484) -> (→"K-2420 2":cluster{"Resistance":sgl})  [unwired: 1 in]
                n148 = Number To Engineering String(2:w483, 3:w483, 4:w484) -> (0:w478:string)  [unwired: 1 in]
                n149 = Bundle(w479, "VISA resource name out"=w486, "error out"=w485) -> (w480:T17)  [unwired: 1 in]
              }
              frame "K-2420 Apply bias" {
                w497 = u16 0 items=["Voltage", "Current"] ("Source Mode  (0: Voltage)")
                w498 = i16 15 ("width (-)")
                n150 = call "Configure Output.vi"("Source Mode  (0: Voltage)"=w497, "error in (no error)"=w493, "Output Level (0)"=w489, "VISA resource name"=w494) -> ("error out"=w495:errorcluster, "VISA resource name out"=w496:refnum<visa-resource-name>)  [unwired: 6 in]
                n151 = call-poly "Read.vi"("VISA resource name"=w496, "error in (no error)"=w495) -> ("VISA resource name out"=w500:refnum<visa-resource-name>, "error out"=w499:errorcluster)  [unwired: 7 in, 5 out]
                n152 = Bundle("Bias (V)"=w489) -> (→"K-2420 4":cluster{"Bias (V)":dbl})  [unwired: 1 in]
                n153 = Number To Engineering String(2:w498, 3:w498, 4:w489) -> (0:w490:string)  [unwired: 1 in]
                n154 = Bundle(w492, "VISA resource name out"=w500, "error out"=w499) -> (w491:T17)  [unwired: 1 in]
              }
            }
          }
        }
        n155 = Unbundle(w361) -> ("Valve position (%)"=w360:dbl, "read pressure"=w355:dbl, "read vapor flow"=w359:dbl, "read gas flow"=w358:dbl)
        n156 = Unbundle("Data logging settings") -> ("Save during sequence only"=w430:bool, "Save now"=w432:bool, "sec between points"=w419:dbl, "Save sample/gas names"=w301:T35)  [unwired: 2 out]
        n157 = property on="Valve position (%)" class="DigNum (strict)"("Value"=w360) -> ()  [unwired: 2 in, 2 out]
        n158 = And(x=w310, y=w430) -> (x .and. y?=w429:bool)
        n159 = Subtract(x=w417, y=w399) -> (x-y=w416:dbl)
        n160 = Bundle("read pressure"=w355) -> (→"pressure chart":cluster{"read pressure":dbl})  [unwired: 1 in]
        n161 = property on="read pressure" class="DigNum (strict)"("Value"=w355) -> ()  [unwired: 2 in, 2 out]
        n162 = Or(x=w429, y=w432) -> (x .or. y?=w426:bool)
        "saving data?" <- w426
        n163 = case shown="True" w331 {
          tunnel: w342 -> [w502 w505]
          tunnel: w341 -> [w501 w506]
          tunnel: [w502 w504] -> w339
          tunnel: [w501 w503] -> w340
          frame False {
          }
          frame True {
            n164 = Concatenate Strings("#000TMPOFF" ("write buffer 2"), "\r", "\n") -> (w507:string)
            n165 = VISA Write(VISA resource name=w505, write buffer=w507, error in (no error)=w506) -> (VISA resource name out=w504:refnum<visa-resource-name>, error out=w503:errorcluster)  [unwired: 1 out]
          }
        }
        n166 = Divide(x=w416, y=60.0) -> (x/y=w391:dbl)
        n167 = property on="read vapor flow" class="DigNum (strict)"("Value"=w359) -> ()  [unwired: 2 in, 2 out]
        n168 = Multiply(x=w419, y=u32 1000 ("x")) -> (x*y=w447:dbl)
        n169 = Bundle("String data out"=w398, w410, w319, w409) -> (w404:T36)  [unwired: 1 in]
        n170 = Wait (ms)(milliseconds to wait=w447) -> ()  [unwired: 1 out]
        n171 = property on="read gas flow" class="DigNum (strict)"("Value"=w358) -> ()  [unwired: 2 in, 2 out]
        n172 = call "data_headers_Jan2017.vi"("Experiment Notes"=w302, "Sample names"=w301) -> ("data headers"=w300:string[])  [unwired: 9 in]
        n173 = Get Date/Time In Seconds() -> (seconds since 1Jan1904=w465:timestamp)
        n174 = Number To Engineering String ("elapsed time (min)")(4:w391) -> (0:w396:string)  [unwired: 3 in]
        n175 = Unbundle(w373) -> ("current  step # in"=w353:i32, "sequence end time in"=w372:timestamp, "Boolean"=w371:bool)
        n176 = Format Date/Time String(time format string (%c)="%Y-%m-%d %H:%M:%S%2u", seconds (now)=w465) -> (date/time string=w444:string)  [unwired: 1 in]
        n177 = Unbundle(w292) -> ("String"=w291:string, "String"=w290:string, "String"=w289:string, "String"=w288:string, "String"=w287:string, "String"=w286:string)
        n178 = Unbundle(w404) -> ("String data out"=w395:string, w394:string, w393:string, w392:string)
        n179 = Unbundle(w443) -> ("String"=w397:string, "String"=w446:string, "String"=w445:string)
        n180 = Unbundle(w388) -> ("String"=w387:string, "String"=w386:string)
        n181 = Unbundle(w362) -> ("pressure"=w442:string, "RH"=w441:string, "gas flow"=w440:string, "vapor flow"=w439:string)
        n182 = Increment(x=w353) -> (x+1=w352:i32)
        n183 = Build Array(w444, w396, w395, w394, w393, w392, w397, w446, w445, w387, w386, w442, w441, w440, w439, w351, w291, w290, w289, w288, w287, w286) -> (w452:string[])
        n184 = property on="Current\nstep" class="DigNum (strict)"("Value"=w352) -> ()  [unwired: 2 in, 2 out]
        "State date/time" <- w390
      }
      n185 = Unbundle(w90) -> (w89:bool, "VISA resource name out"=w88:refnum<visa-resource-name>, "error out"=w87:errorcluster)
      n186 = Unbundle(w86) -> ("Boolean"=w85:bool, "VISA out"=w84:refnum<visa-resource-name>, "error out"=w83:errorcluster)
      n187 = call-poly <vilib>:"Write To Spreadsheet File.vi"("1D data"=w55, "file path (dialog if empty)"=w71) -> ("new file path (Not A Path if cancelled)"=w75:path)  [unwired: 6 in]
      n188 = Unbundle(w64) -> (w69:bool, "VISA resource name out"=w68:refnum<visa-resource-name>, "error out"=w67:errorcluster)
      n189 = Unbundle(w37) -> ("Boolean"=w36:bool, "task out"=w19:refnum<k21>, "error out"=w18:errorcluster, "task out"=w17:refnum<k21>, "error out"=w16:errorcluster, "VISA resource name out"=w15:refnum<visa-resource-name>, "error out"=w14:errorcluster)
      n190 = call "arduino_close_subIV.vi"("arduino 1-6 addresses and errors out"=w57, "arduinos on?"=w56) -> ()  [unwired: 10 in]
      n191 = case shown="True" w49 {
        tunnel: w48 -> [_ w110]
        tunnel: w47 -> [w107 w109]
        tunnel: [w107 w108] -> w46
        frame False {
        }
        frame True {
          n192 = call "Close.vi"("VISA resource name"=w110, "error in (no error)"=w109) -> ("error out"=w108:errorcluster)  [unwired: 17 in]
        }
      }
      n193 = flat-sequence {
        tunnel: w24 -> [w106]
        tunnel: [w106] -> w23
        frame #0 {
          n194 = property on="saving data?" class="Bool (strict)"("Value"=FALSE ("saving data?")) -> ()  [unwired: 2 in, 2 out]
        }
      }
      n195 = Unbundle(w81) -> ("Boolean"=w80:bool, "VISA resource name out"=w79:refnum<visa-resource-name>, "error out"=w78:errorcluster)
      n196 = case shown="True" w36 {
        tunnel: [errorcluster {"status"=FALSE, "code"=0, "source"=""} ("error out") w135] -> w41
        tunnel: w19 -> [_ w134]
        tunnel: w18 -> [_ w133]
        tunnel: w17 -> [_ w132]
        tunnel: w16 -> [_ w129]
        tunnel: w15 -> [_ w130]
        tunnel: w14 -> [_ w131]
        tunnel: w10 -> [_ w126]
        tunnel: w9 -> [_ w125]
        frame False {
        }
        frame True {
          n197 = call <vilib>:"DAQmx Stop Task.vi"("task/channels in"=w134, "error in"=w133) -> ("task out"=w141:refnum<k21>, "error out"=w140:errorcluster)  [unwired: 12 in]
          n198 = call <vilib>:"DAQmx Stop Task.vi"("task/channels in"=w132, "error in"=w129) -> ("task out"=w142:refnum<k21>, "error out"=w143:errorcluster)  [unwired: 12 in]
          n199 = VISA Clear(VISA resource name=w130, error in (no error)=w131) -> (VISA resource name out=w139:refnum<visa-resource-name>, error out=w138:errorcluster)
          n200 = VISA Close(VISA resource name=w126, error in (no error)=w125) -> (error out=w127:errorcluster)
          n201 = VISA Close(VISA resource name=w139, error in (no error)=w138) -> (error out=w128:errorcluster)
          n202 = call <vilib>:"DAQmx Clear Task.vi"("task in"=w141, "error in"=w140) -> ("error out"=w137:errorcluster)  [unwired: 13 in]
          n203 = call <vilib>:"DAQmx Clear Task.vi"("task in"=w142, "error in"=w143) -> ("error out"=w136:errorcluster)  [unwired: 13 in]
          n204 = Merge Errors(w137, w136, w128, w127) -> (w135:errorcluster)
        }
      }
      n205 = case shown="True" w89 {
        tunnel: w88 -> [_ w260]
        tunnel: w87 -> [w257 w259]
        tunnel: [w257 w258] -> w91
        frame False {
        }
        frame True {
          n206 = call "Enable Output.vi"("error in (no error)"=w259, "Enable Output (T: Enable)"=FALSE, "VISA resource name"=w260) -> ("error out"=w261:errorcluster, "VISA resource name out"=w263:refnum<visa-resource-name>)  [unwired: 7 in]
          n207 = call "Close.vi"("error in (no error)"=w261, "VISA resource name"=w263) -> ("error out"=w258:errorcluster)  [unwired: 9 in]
        }
      }
      n208 = case shown="True" w69 {
        tunnel: w68 -> [_ w174]
        tunnel: w67 -> [w172 w173]
        tunnel: [w172 w175] -> w63
        frame False {
        }
        frame True {
          n209 = call "Enable Output.vi"("error in (no error)"=w173, "Enable Output (F:Off)"=FALSE ("Output (F:Off)"), "VISA resource name"=w174) -> ("error out"=w176:errorcluster, "VISA resource name out"=w177:refnum<visa-resource-name>)  [unwired: 7 out]
          n210 = call "Close.vi"("error in (no error)"=w176, "VISA resource name"=w177) -> ("error out"=w175:errorcluster)  [unwired: 9 out]
        }
      }
      n211 = case shown="True" w85 {
        tunnel: w83 -> [w243 w246]
        tunnel: [w243 w245] -> w92
        tunnel: w84 -> [_ w244]
        frame False {
        }
        frame True {
          n212 = call "srsQcm200Close.vi"("error in"=w246, "Visa in"=w244) -> ("error out"=w245:errorcluster)  [unwired: 3 in]
        }
      }
      n213 = call-poly <vilib>:"Write To Spreadsheet File.vi"("append to file? (new file:F)"=TRUE, "2D data"=w59, "file path (dialog if empty)"=w75) -> ()  [unwired: 5 in, 1 out]
      n214 = case shown="True" w80 {
        tunnel: w79 -> [_ w213]
        tunnel: w78 -> [w210 w212]
        tunnel: [w210 w211] -> w77
        frame False {
        }
        frame True {
          n215 = VISA Close(VISA resource name=w213, error in (no error)=w212) -> (error out=w211:errorcluster)
        }
      }
      n216 = Merge Errors(w63, w77, w91, w46, w92, w23) -> (w98:errorcluster)
      n217 = call <vilib>:"Simple Error Handler.vi"("error in (no error)"=w41) -> ()  [unwired: 4 in, 5 out]
      n218 = call <vilib>:"Simple Error Handler.vi"("error in (no error)"=w98) -> ()  [unwired: 4 in, 5 out]
    }
  }
